vi "Type.vi"(11 "RelationPanel in":refnum<class "RelationPanel.lvclass">) -> (2 "Type":refnum<class "Type.lvclass">)   [LabVIEW 2020, in "Conditum-Tools.lvlib" / "RelationPanel.lvclass"]
uses:
  RelationPanel.lvclass
  Conditum-Clone/Columns/Type/Type.lvclass
  RelationPanel.lvclass/RelationPanel.ctl
  Conditum-Clone/Columns/Relation/Relation.lvclass
  C:/dev/lv20CE/lv-conditum-tools/Conditum-Clone/Columns/Type/Type.lvclass
  C:/dev/lv20CE/lv-conditum-tools/Conditum-Clone/Columns/Relation/Relation.lvclass
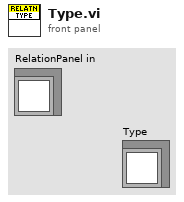
[diagram p1: front panel]
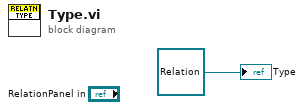
[diagram p0: block diagram]
diagram:
  "Type" <- refnum<class "Relation.lvclass"> refnum ("Conditum:Columns:Relation.lvclass")
